vi "A.vi"(2 "積木種類":enum16{"0", "1", "2", "3", "4", "5", "6"}(ring), 3 "初始進入":bool[][](array[boolean]), 8 "KNR in 2":T1, 9 "Error":errorcluster) -> (0 "旋轉數":i32, 5 "底盤T數":i32, 10 "KNR out":T1, 11 "error out":errorcluster, 14 "end":i32, 15 "Y軸補正":i32, 16 "移動位置":i32, 17 "最終堆疊版":bool[][](array[boolean]), 19 "層數":i32)   [LabVIEW 2013]
uses:
  <userlib>/KNR OS 3.0 LabVIEW Toolkit/Type Definition/KNR3 Reference.ctl
  <userlib>/_FPGA Interface Advanced Tools/FPGA Interface Base/FPGA Interface Base.lvclass
  <userlib>/KNR OS 3.0 LabVIEW Toolkit/Type Definition/Resource.ctl
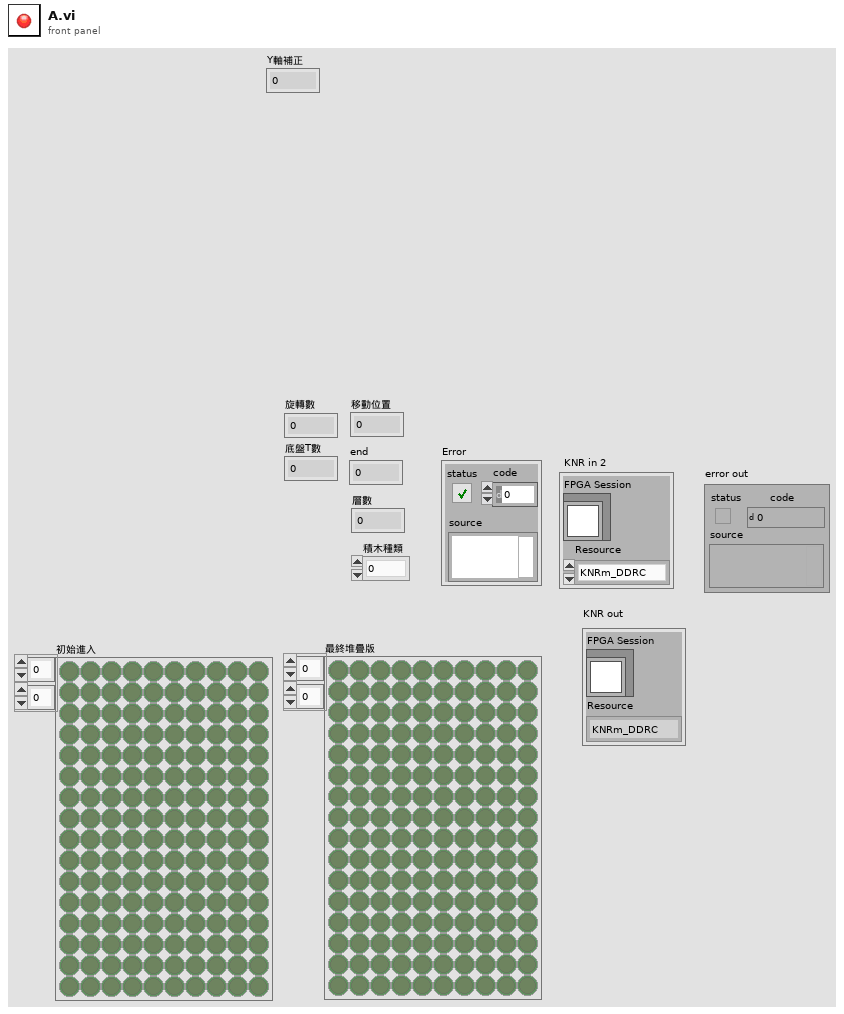
[diagram p1: front panel]
types:
  T1 = typedef "KNR3 Reference.ctl" = cluster{"FPGA Session":refnum<class "FPGA Interface Base.lvclass">, "Resource":T2}
  T2 = typedef "Resource.ctl" = enum16{"KNRm_DDRC", "KNRm_DDDD", "KNRm_DDDR", "KNRm_DDDC", "KNR"}
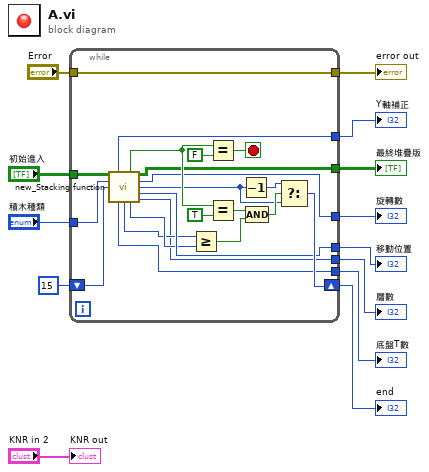
[diagram p0: block diagram]
diagram:
  n1 = while {
    tunnel: "初始進入" -> [w25]
    tunnel: [w27] -> w12
    tunnel: "積木種類" -> [w24]
    shift-right: [w32] -> w8
    shift-left: 15 -> [w26]
    tunnel: [w23] -> w9
    tunnel: "Error" -> [w18]
    tunnel: [w18] -> w6
    tunnel: [w17] -> w4
    tunnel: [w16] -> w3
    tunnel: [w15] -> w2
    tunnel: [w14] -> w1
    stop <- w33 stop-if-true
    n2 = call "new_Stacking function.vi"("初始進入"=w25, "積木種類"=w24, "15"=w26) -> ("Y軸補正"=w14:i32, "匹配位置"=w28:bool, "最終堆疊版"=w27:bool[][], "rolloo"=w16:i32, "end"=w22:i32, "移動位置"=w23:i32, "底盤T數"=w15:i32, "旋轉數"=w19:i32, "roll"=w20:i32, "層數"=w17:i32)  [unwired: 2 in, 1 out]
    n3 = Greater Or Equal?(x=w19, y=w20) -> (x >= y?=w31:bool)
    n4 = Equal?(x=w28, y=FALSE) -> (x = y?=w33:bool)
    n5 = Equal?(x=w28, y=TRUE) -> (x = y?=w29:bool)
    n6 = Decrement(x=w22) -> (x-1=w21:i32)
    n7 = Compound Arithmetic op=AND(w29, w31) -> (w35:bool)
    n8 = Select(t=w21, s=w35, f=w22) -> (s? t:f=w32:i32)
  }
  "最終堆疊版" <- w12
  "移動位置" <- w9
  "end" <- w8
  "error out" <- w6
  "層數" <- w4
  "旋轉數" <- w3
  "底盤T數" <- w2
  "Y軸補正" <- w1
  "KNR out" <- "KNR in 2"
